vi "MOCOAUTOMATION_1.0.vi"() -> ()   [LabVIEW 2009]
uses:
  autostatus.ctl
  DAQGlobal.vi
  global_m.vi
  1608fsdr/Global 3.vi
  Global 2.vi
panel:
  out "GoTo Wavelength":dbl
  out "Waiting on Move":bool
  out "Exposure Time:":dbl
  out "Number of Steps:":dbl
  out "Step Size:":dbl
  out "Min nm":dbl
  out "Max nm":dbl
  in  "Start up Blinking":bool=TRUE
  in  "Delay Before\nread (ms)":u32=50
  out "delay":u16
  out "back_L":bool
  out "Shutter OFF":bool
  out "Shutter ON":bool
  in  "Tab Control":enum32{"Setup", "Operation"}(tab)
  in  "Automation":bool
  in  "Save settings":bool
  in  "Initialize":bool caption="Push at start up"
  in  "Grating, gr/mm":u16(ring)=2 items=["2400", "1800", "1200", "600", "300", "150"]
  in  "Backlash compensation":dbl=10.0 format="%.2f"
  in  "Backlash":bool
  in  "Calibration, nm":dbl=265.0 format="%2.2f"
  in  "Communication port":refnum<visa-resource-name>="COM1"
  out "Shutter":bool
  in  "Sh_OFF":bool
  in  "Sh_ON":bool
  in  "Speed_set":bool
  in  "Speed":dbl=50.0 format="%.3f"
  in  "stop 2":bool
  in  "fs":bool
  in  "bs":bool
  in  "Wavelength, nm":dbl=10.0 format="%.2f"
  in  "GoTo":bool
  in  "Destination Wavelength":dbl=500.0 format="%.2f"
  out "Present Wavelength":dbl format="%.2f"
  out "move done":bool
  out "string 2":string="\n"
  in  "return":bool
  in  "String To Write 3":string="Y-1?"
  out "Loop":i32
  in  "write":bool
  out "command sent":string="\n"
  out "writing":bool
  in  "stop":bool
  out "read string":string="\n"
  # "Backlash \nCompensation, nm"
  # "nm"
  # "Wavelength"
  # "nm"
  # "Move Wavelength"
  # "nm"
  # "nm/sec"
  # "Shutter"
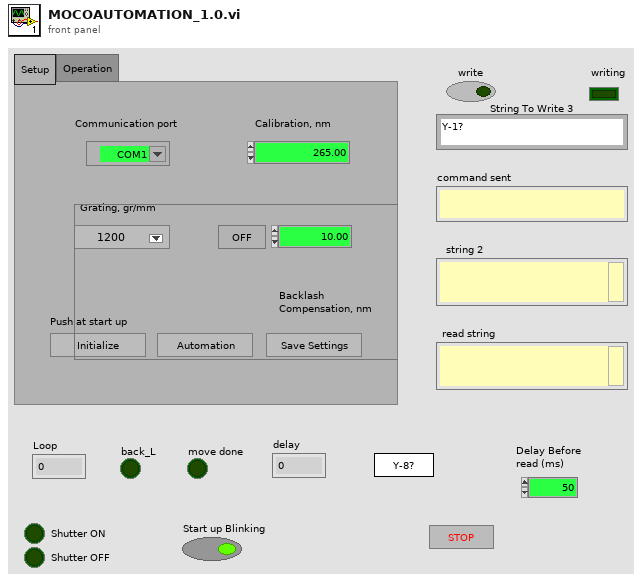
[diagram p1: front panel]
types:
  T1 = enum16{"open", "replace", "create", "open or create", "replace or create", "replace or create with confirmation"}
  T2 = typedef "autostatus.ctl" = enum16{"Default", "Initilize Wavelength", "Shutter Open", "Photodiode Aquire", "Take Img", "Wait Exposure Time", "Photodiode Off", "Shutter Close", "Acquire Dark", "Next Wavelength"}
  T3 = cluster{"Max nm":dbl, "Min nm":dbl, "Step Size:":dbl, "Number of Steps:":dbl, "Exposure Time:":dbl, "Regulation:":bool, "Temperature:":dbl, "Wait_For_Temp:":bool}
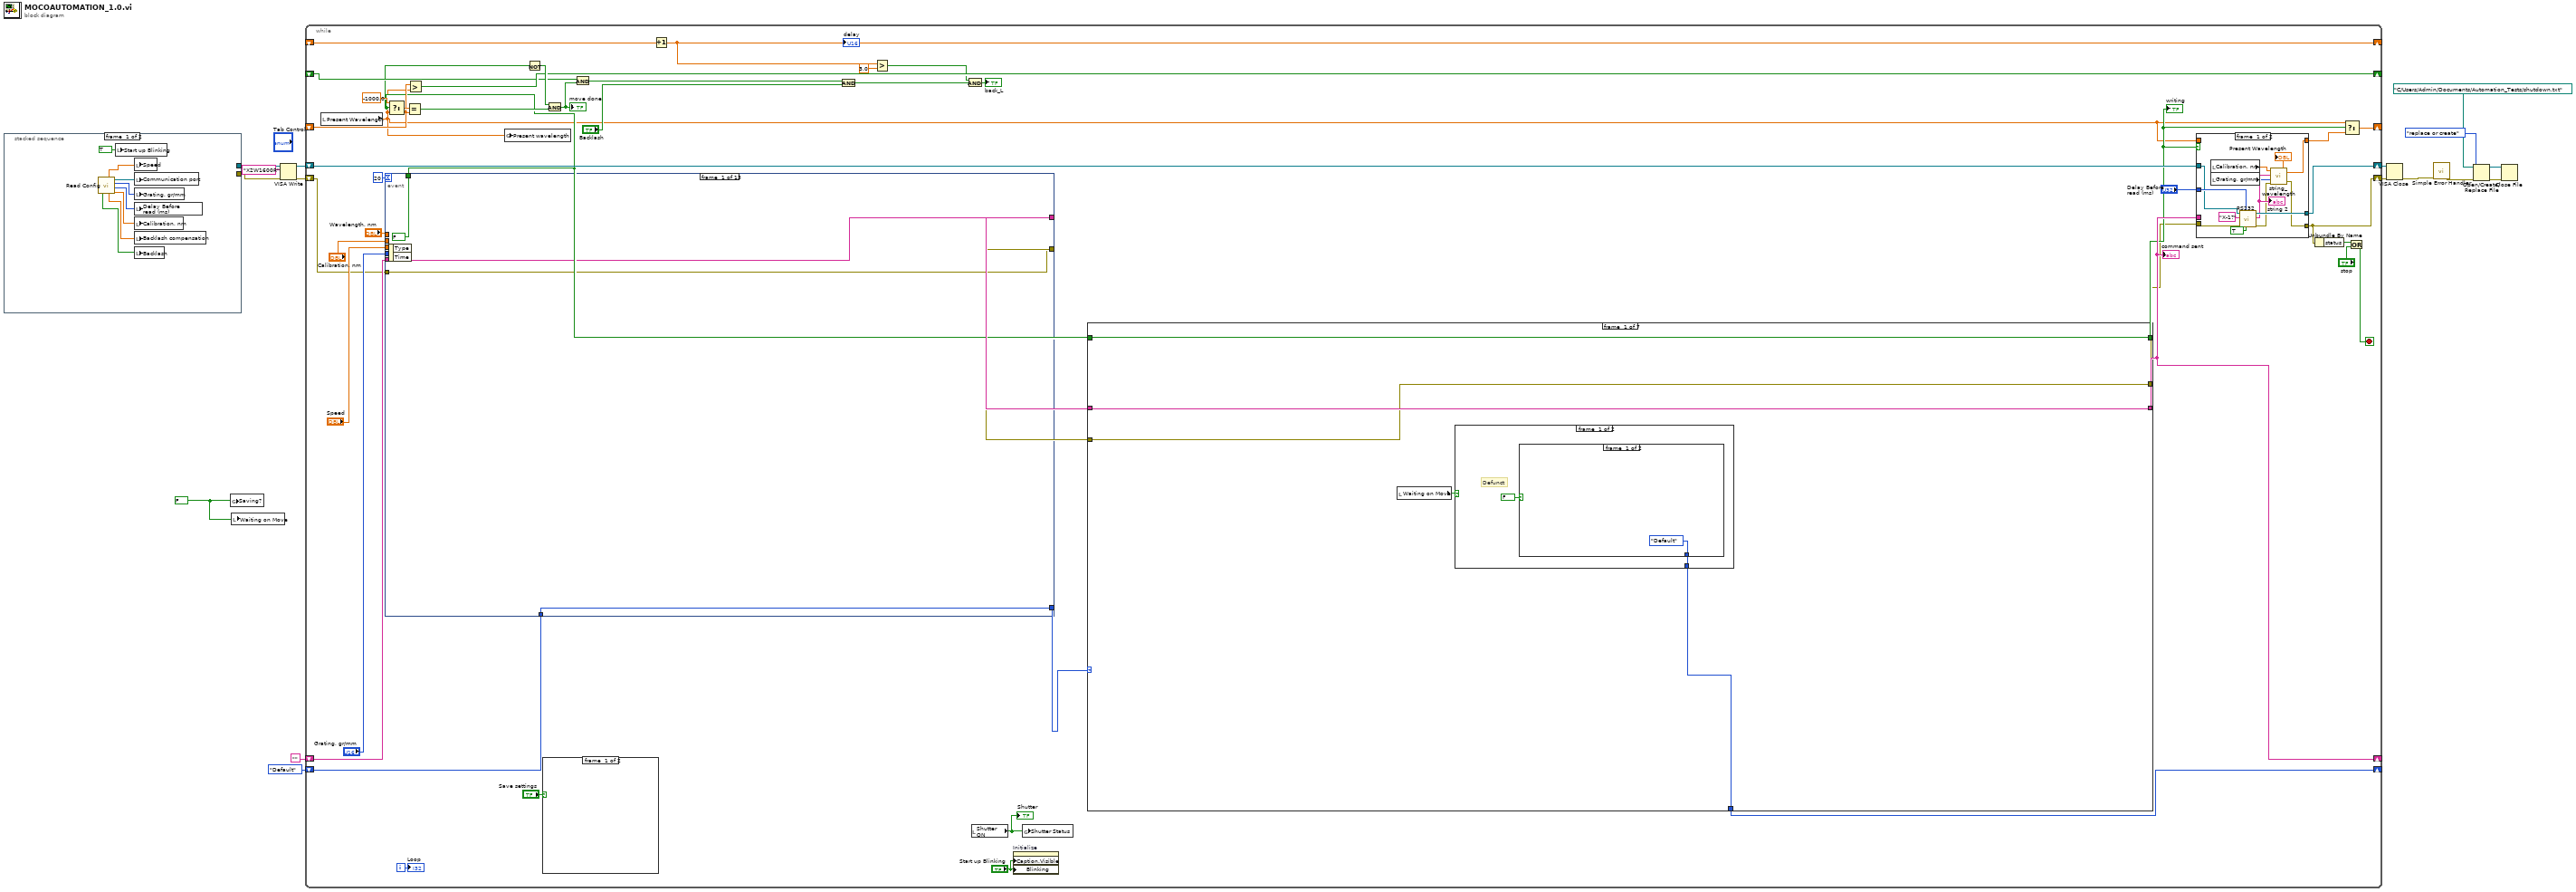
[diagram p0: block diagram]
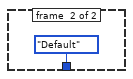
[diagram p2: hidden frame]
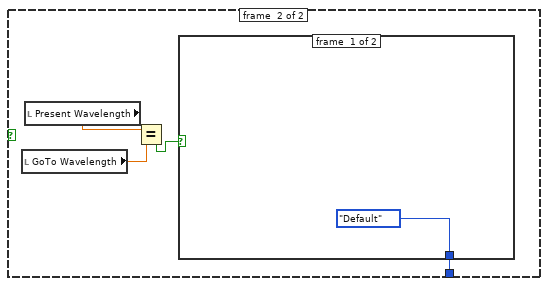
[diagram p3: hidden frame]
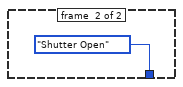
[diagram p4: hidden frame]
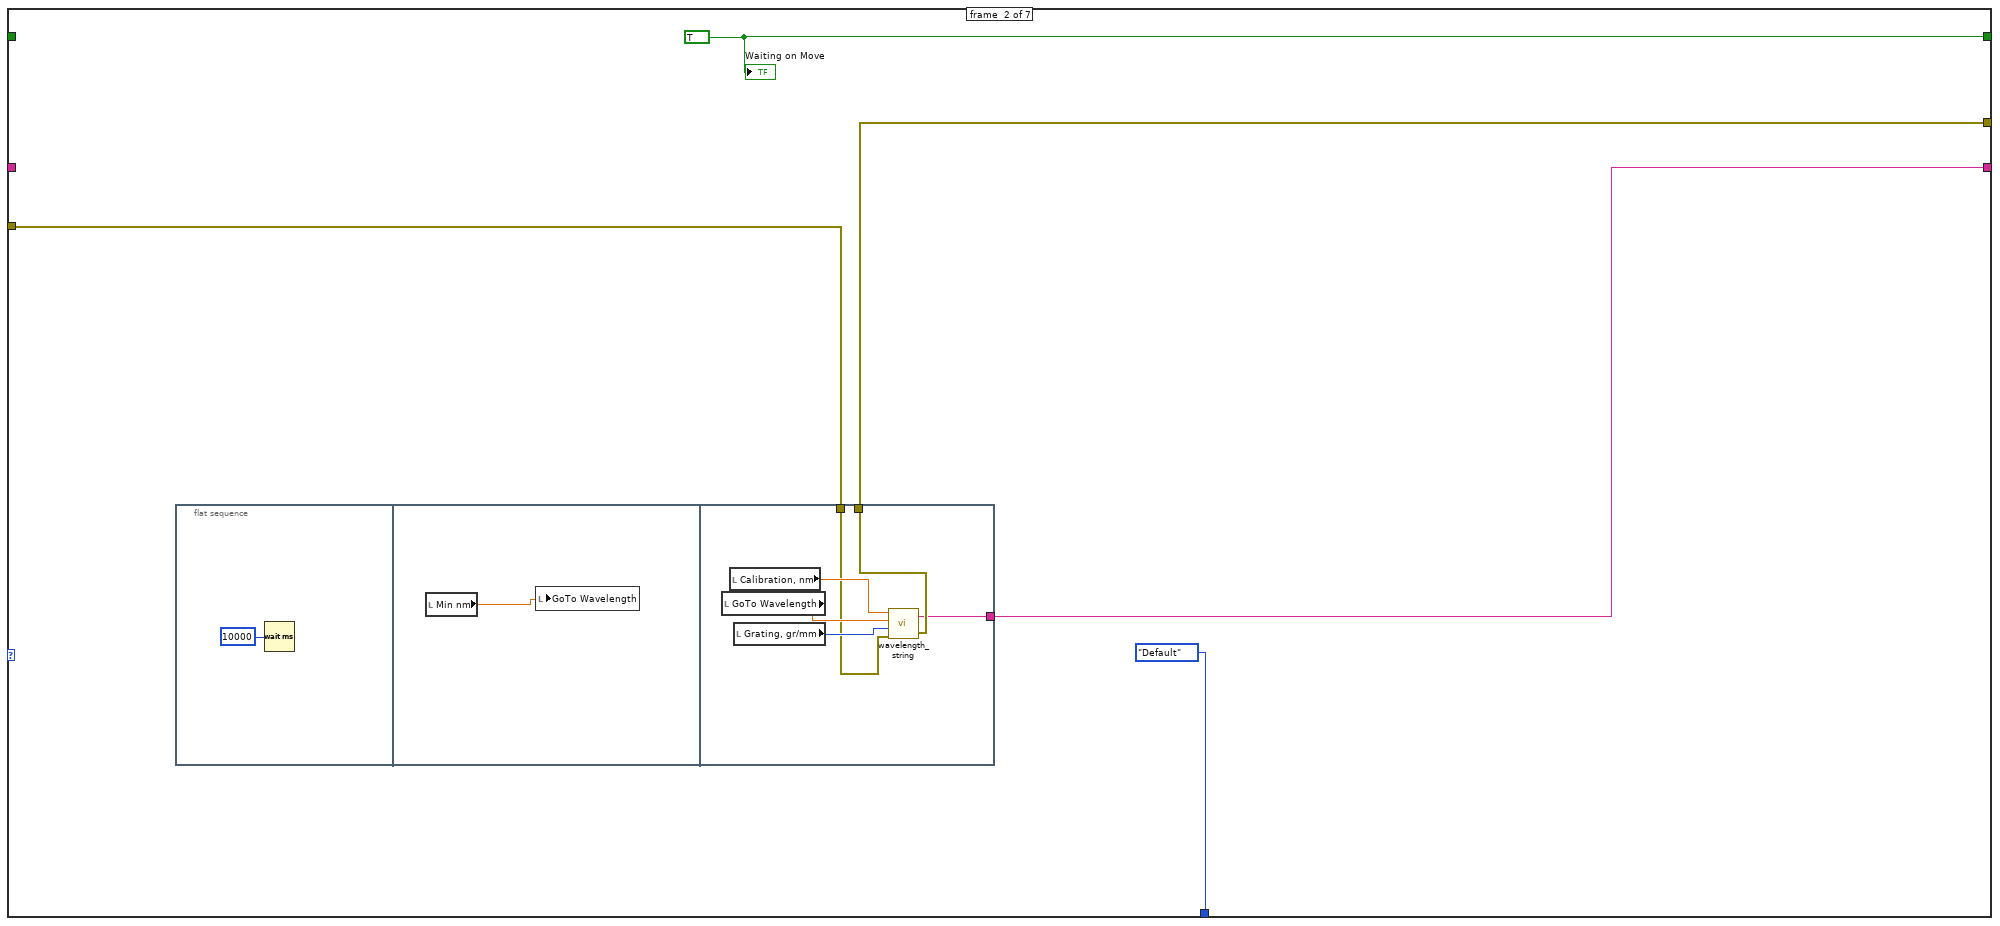
[diagram p5: hidden frame]
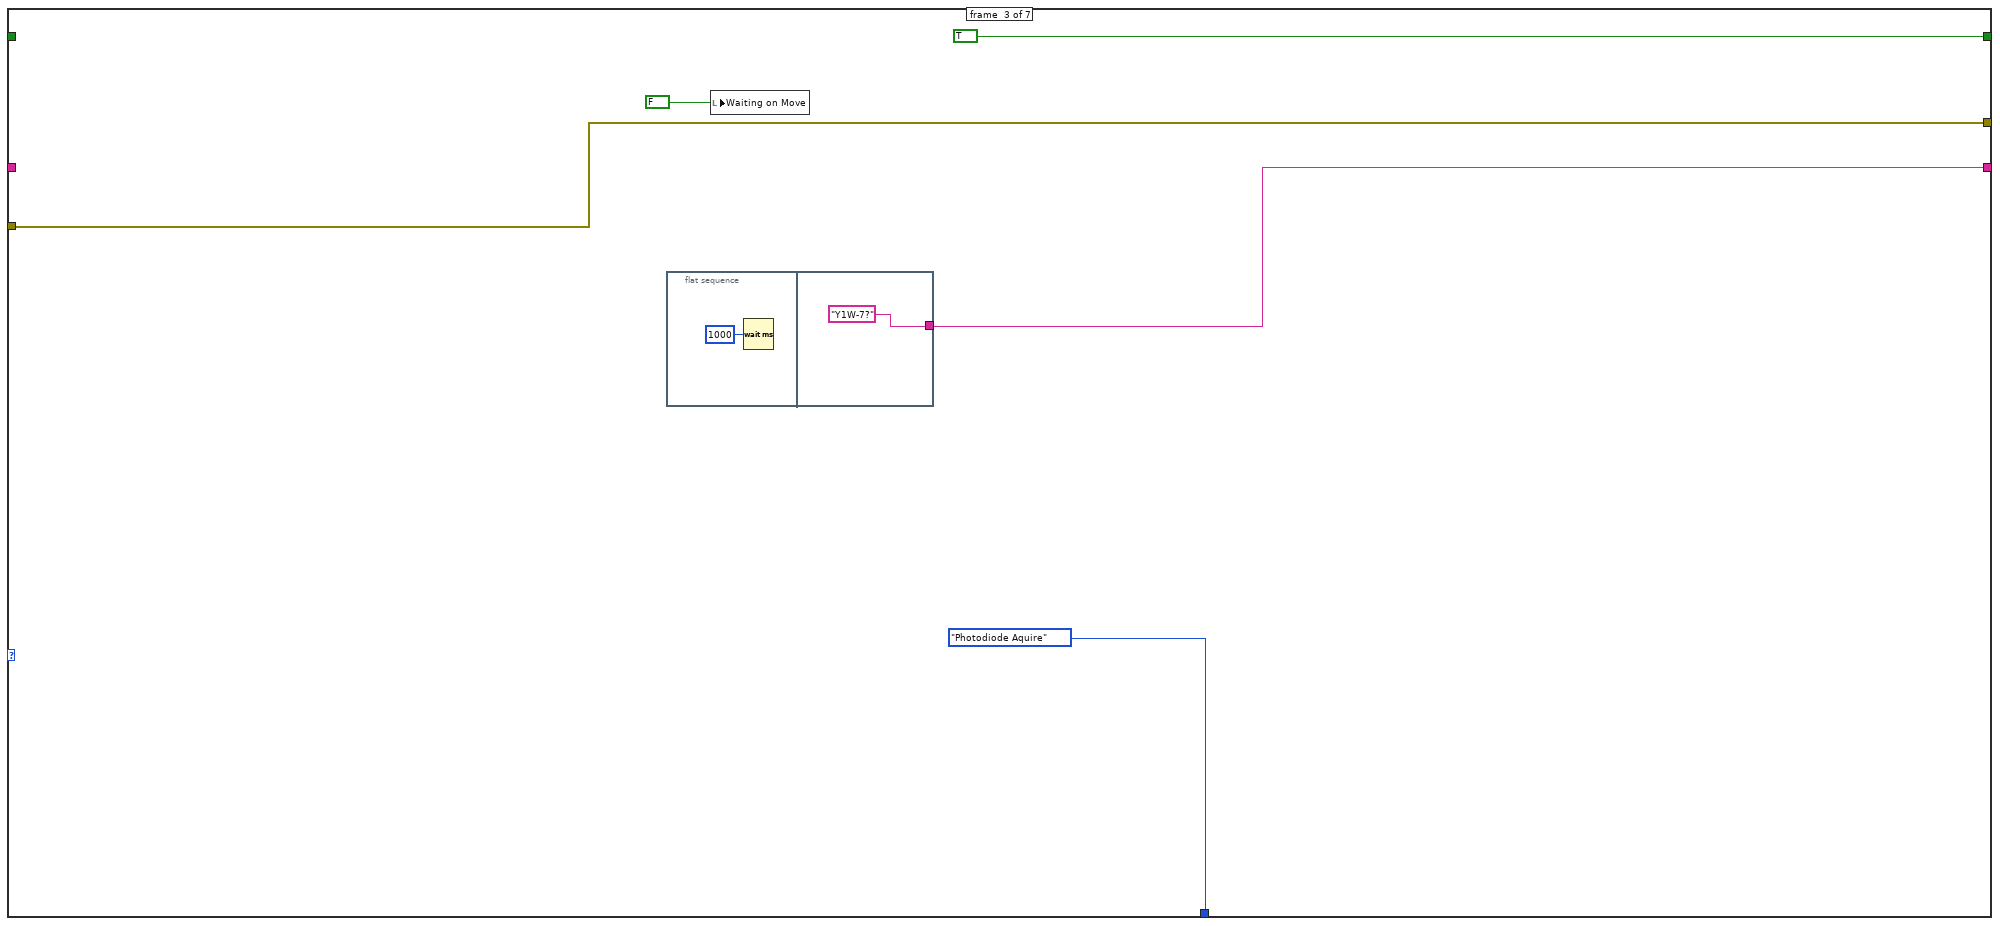
[diagram p6: hidden frame]
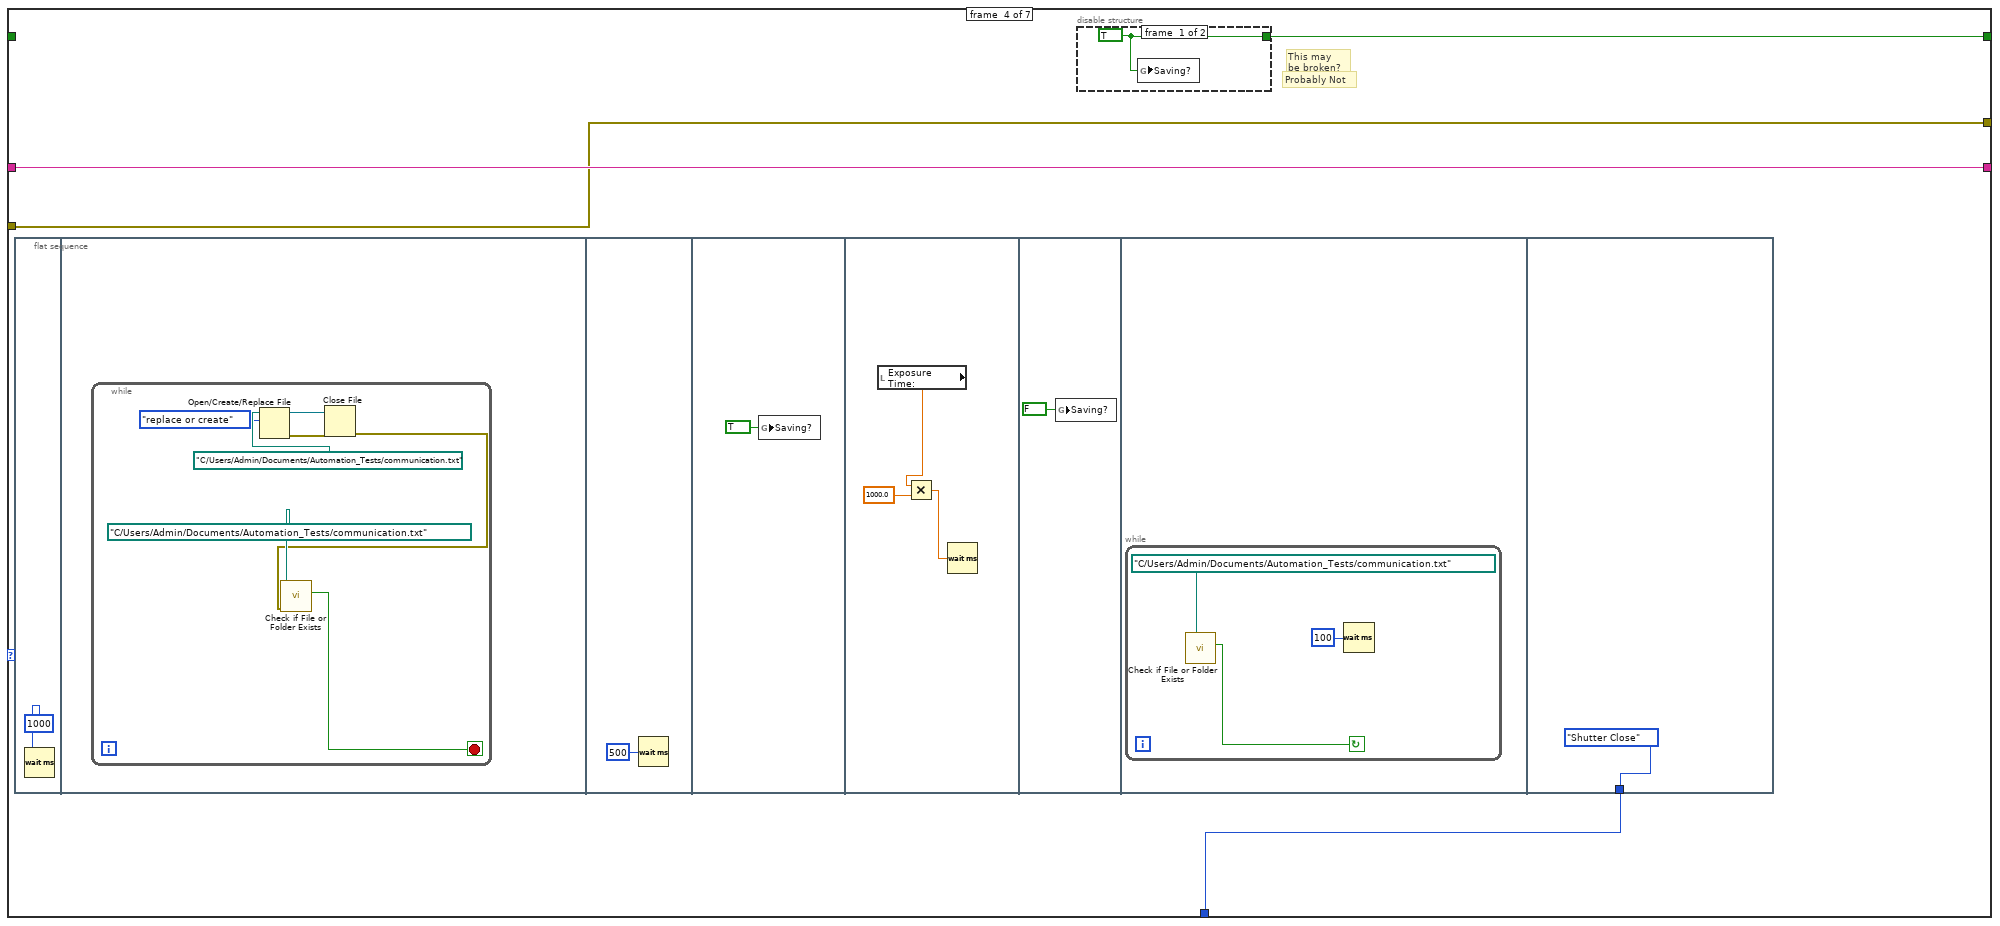
[diagram p7: hidden frame]
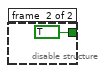
[diagram p8: hidden frame]
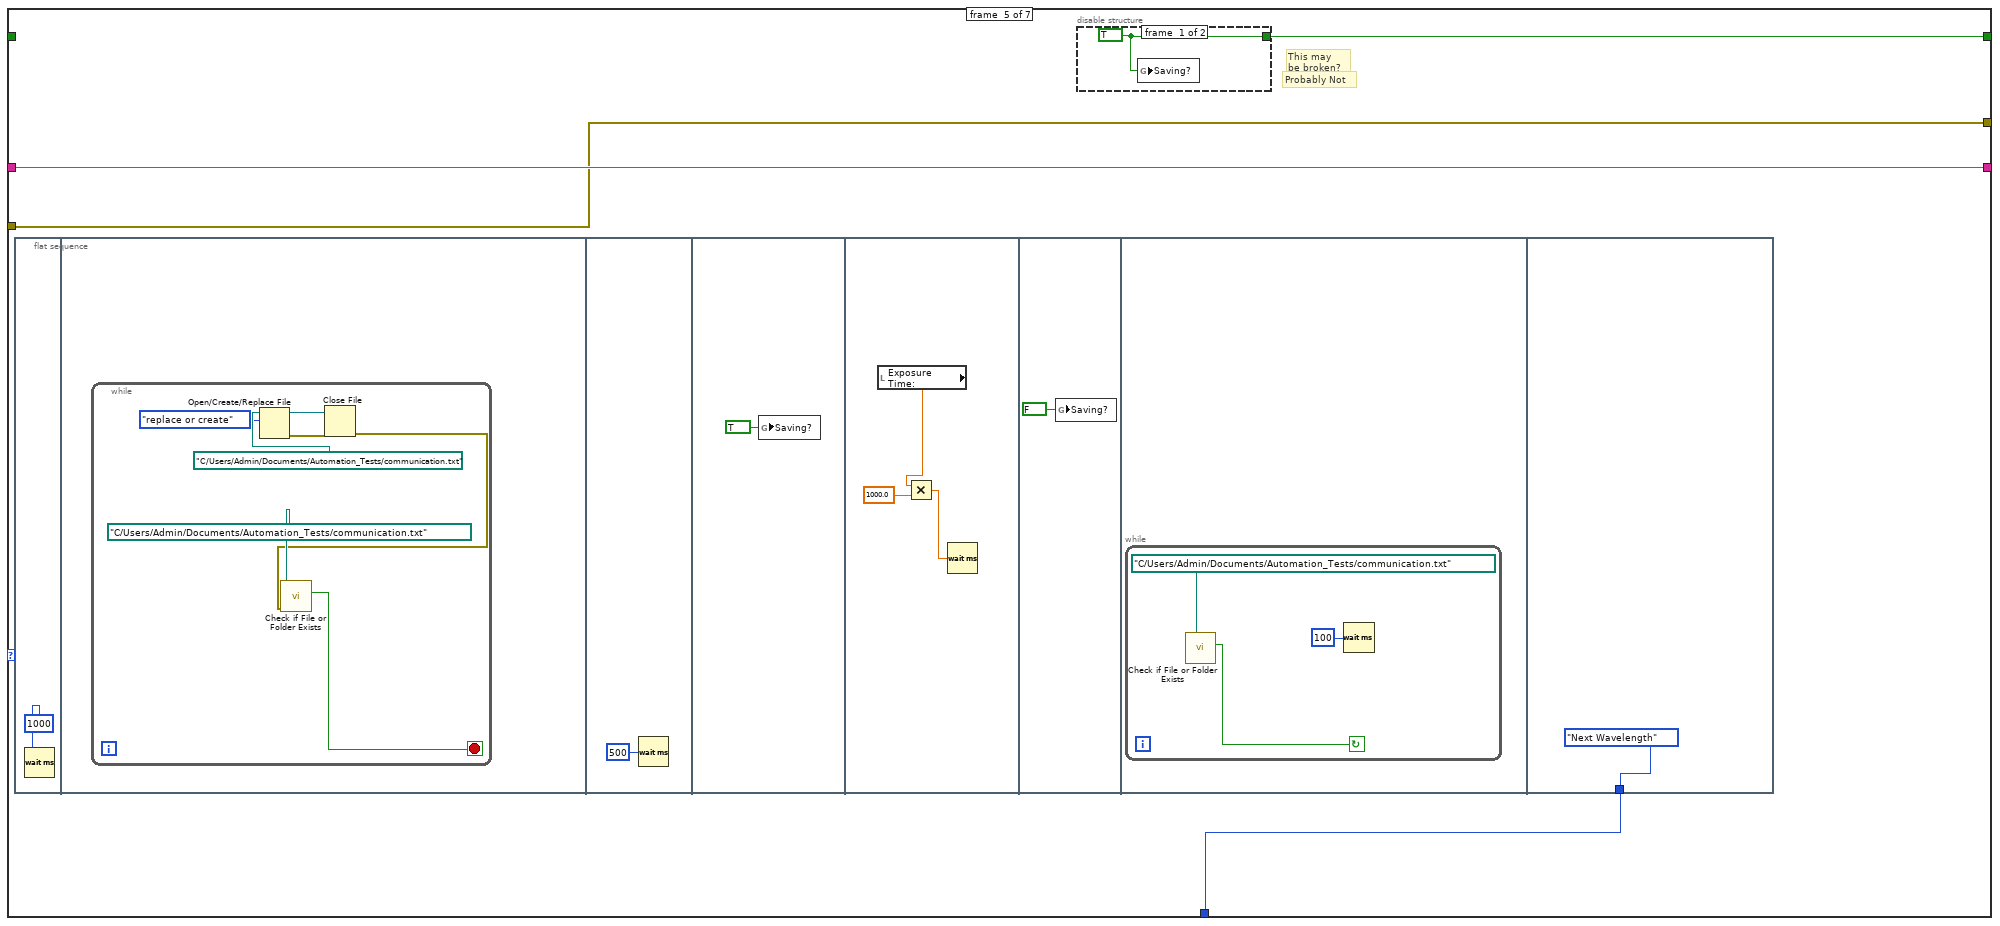
[diagram p9: hidden frame]
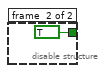
[diagram p10: hidden frame]
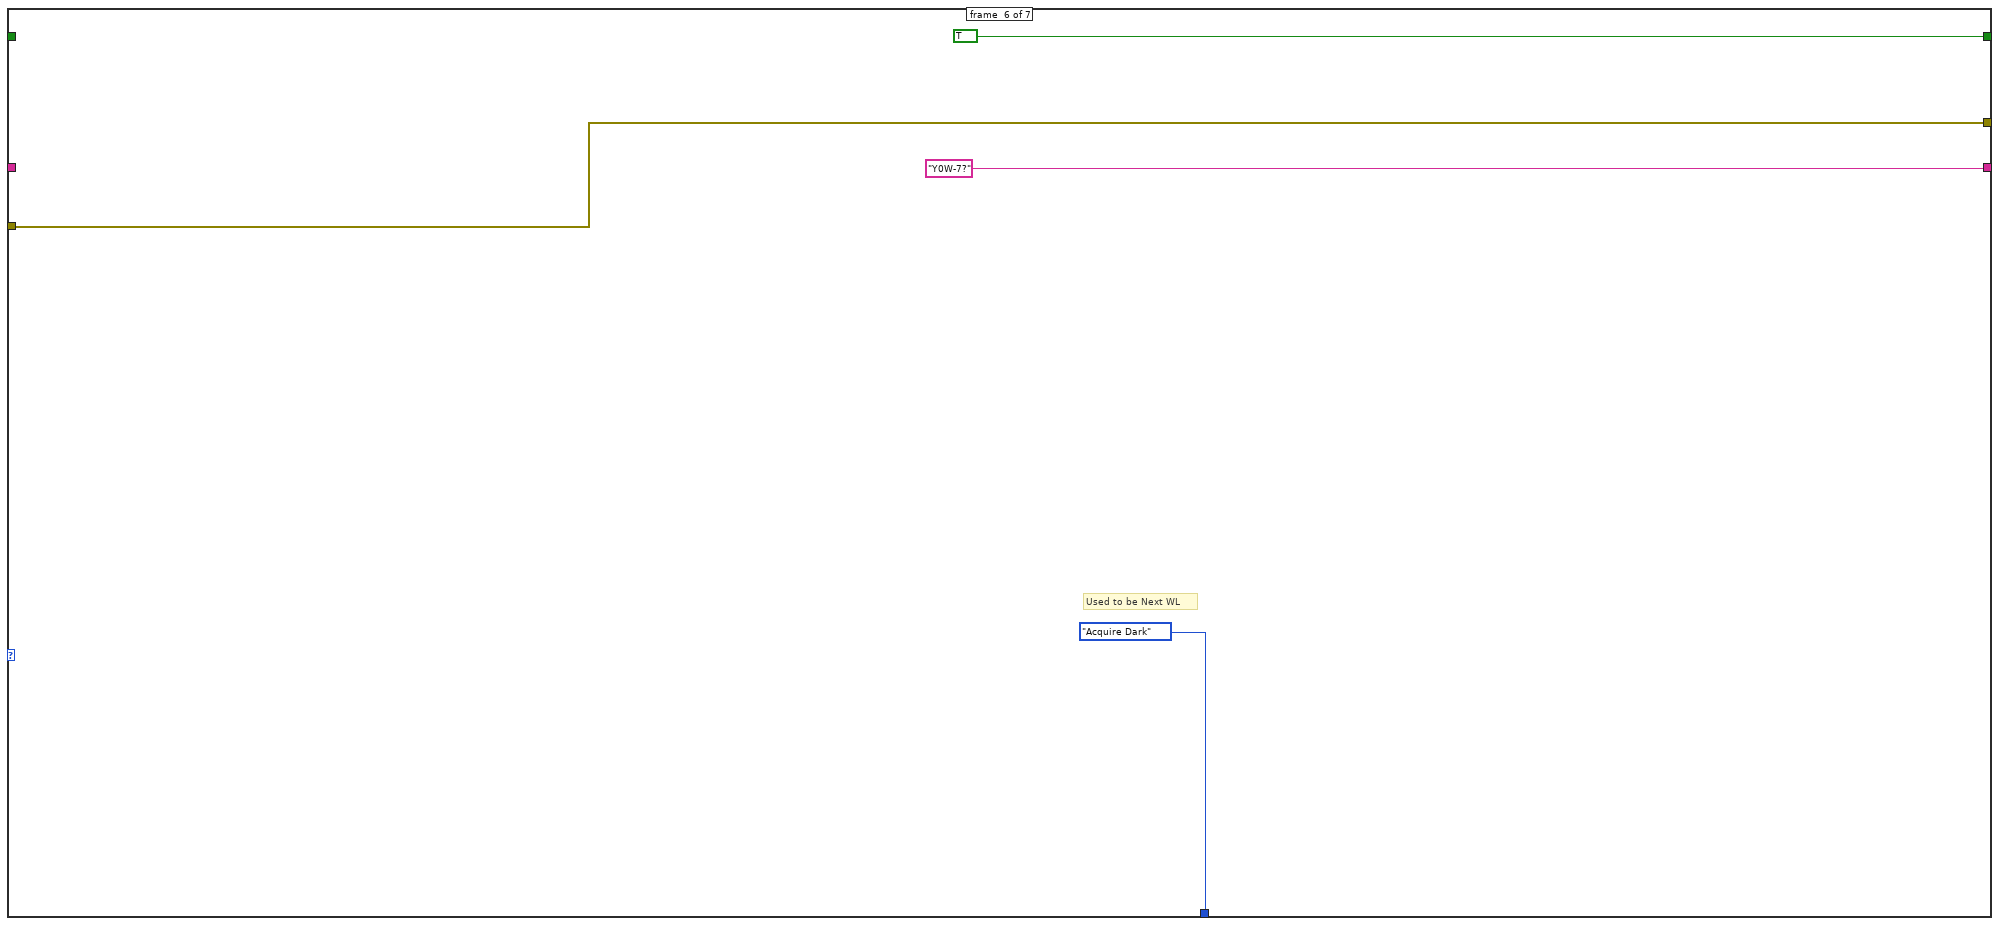
[diagram p11: hidden frame]
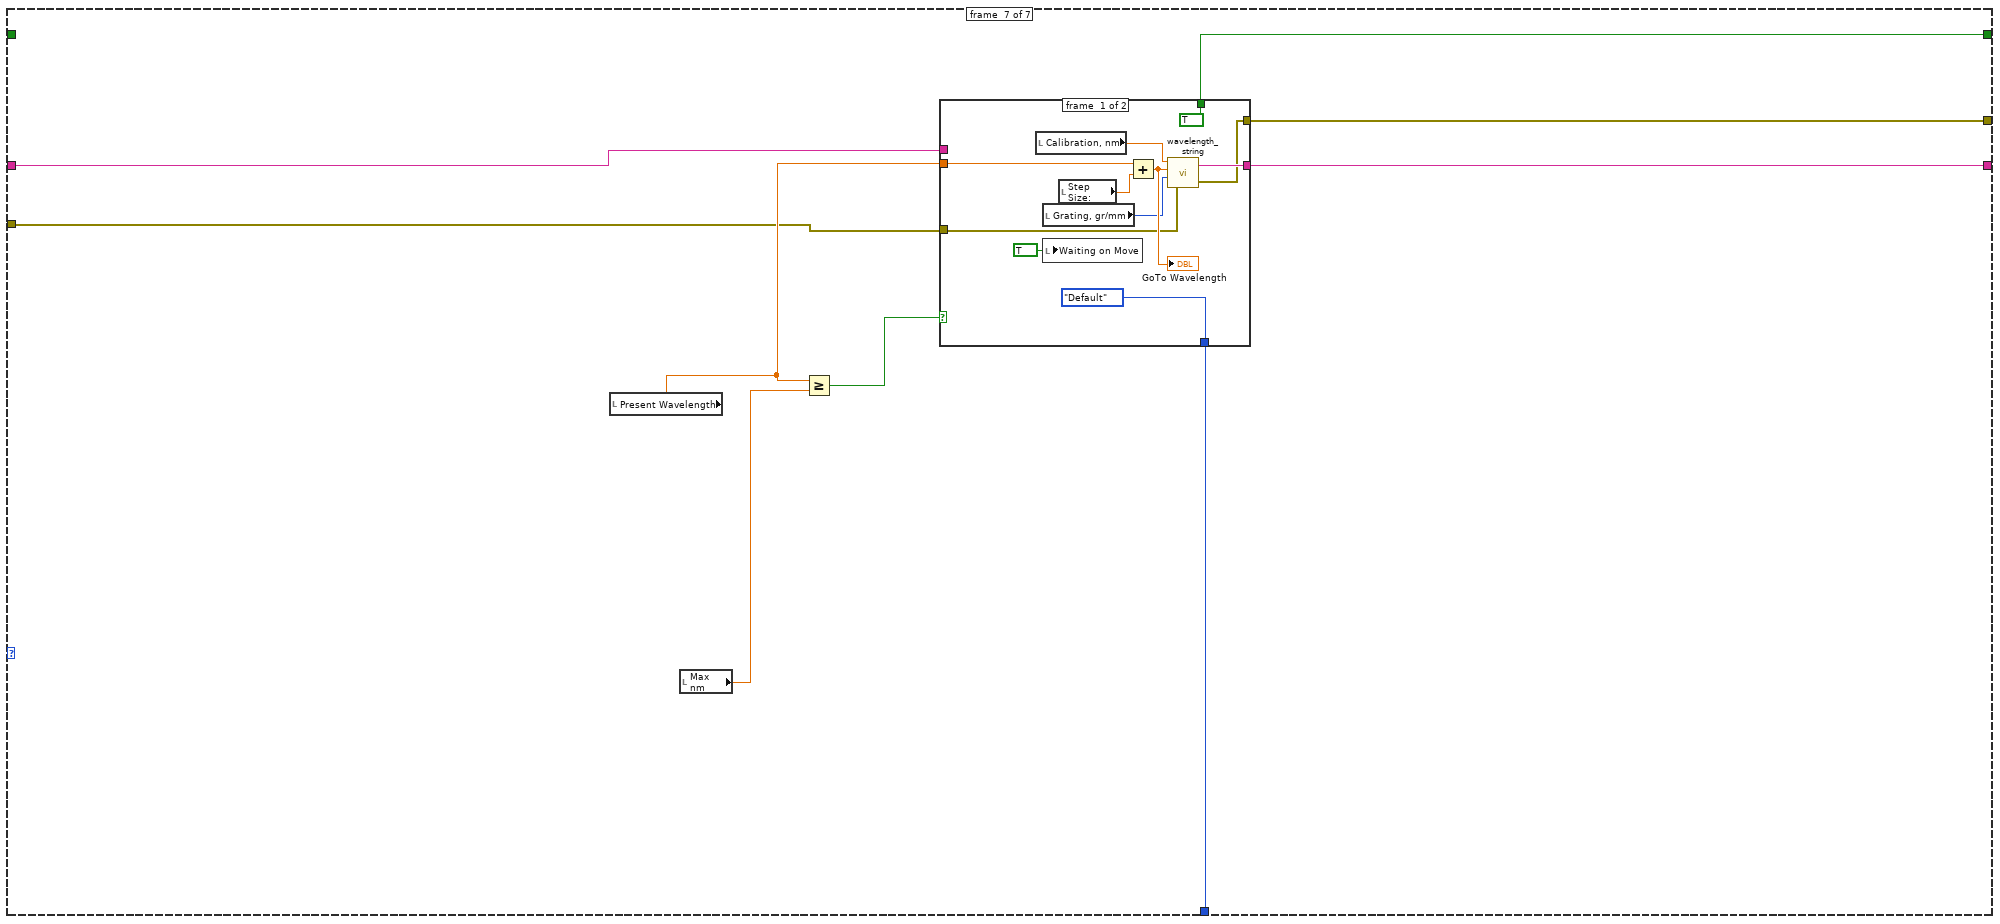
[diagram p12: hidden frame]
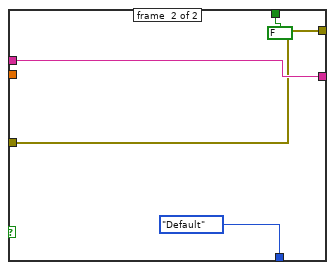
[diagram p13: hidden frame]
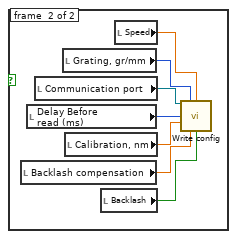
[diagram p14: hidden frame]
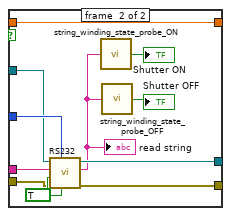
[diagram p15: hidden frame]
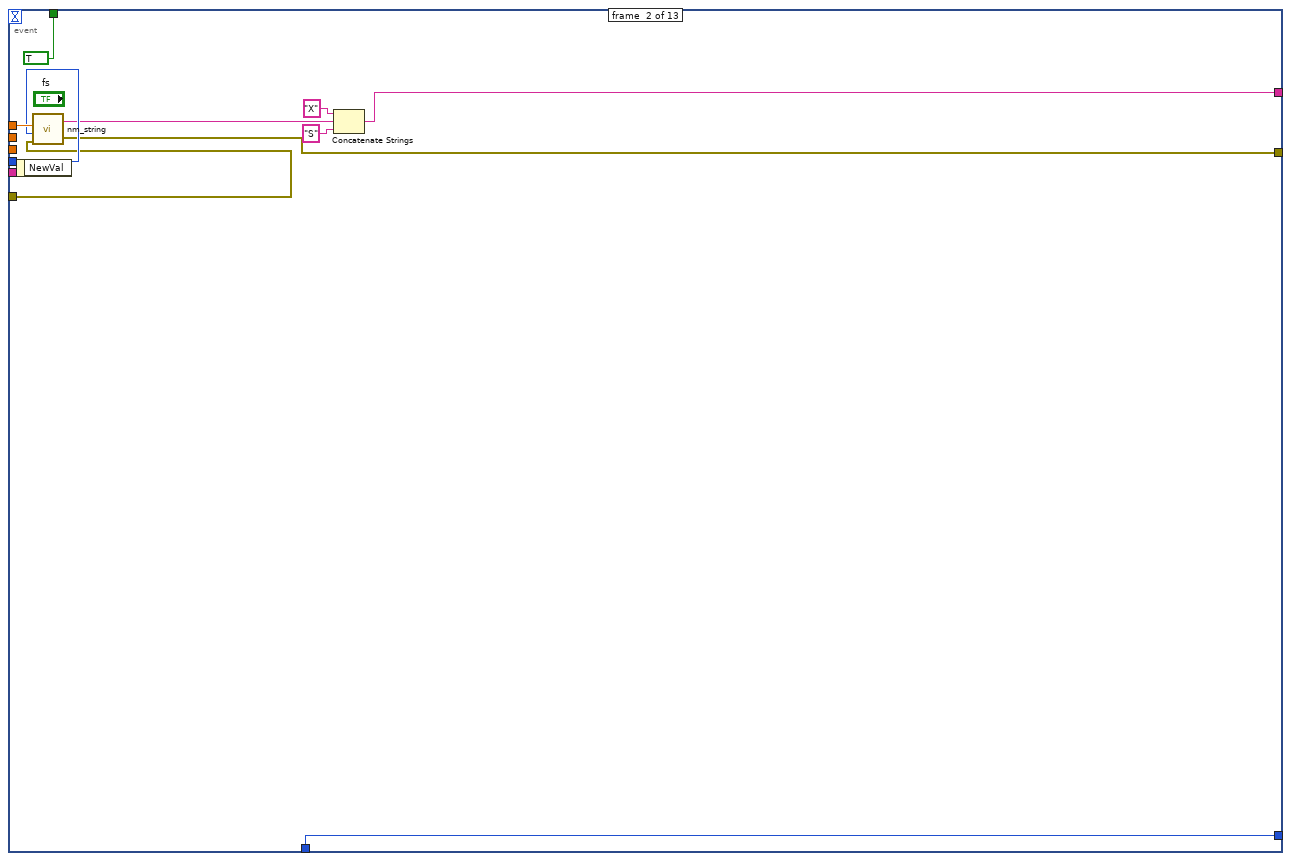
[diagram p16: hidden frame]
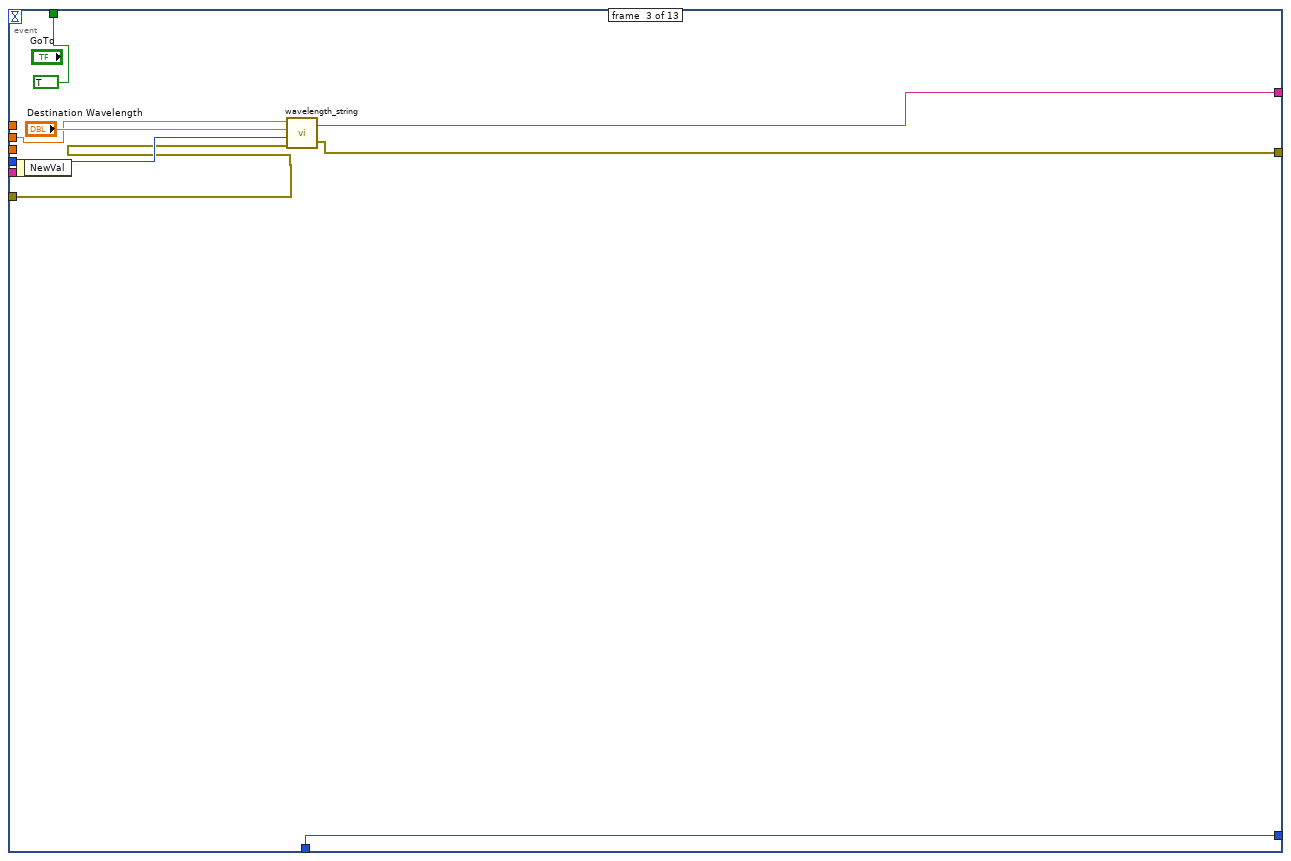
[diagram p17: hidden frame]
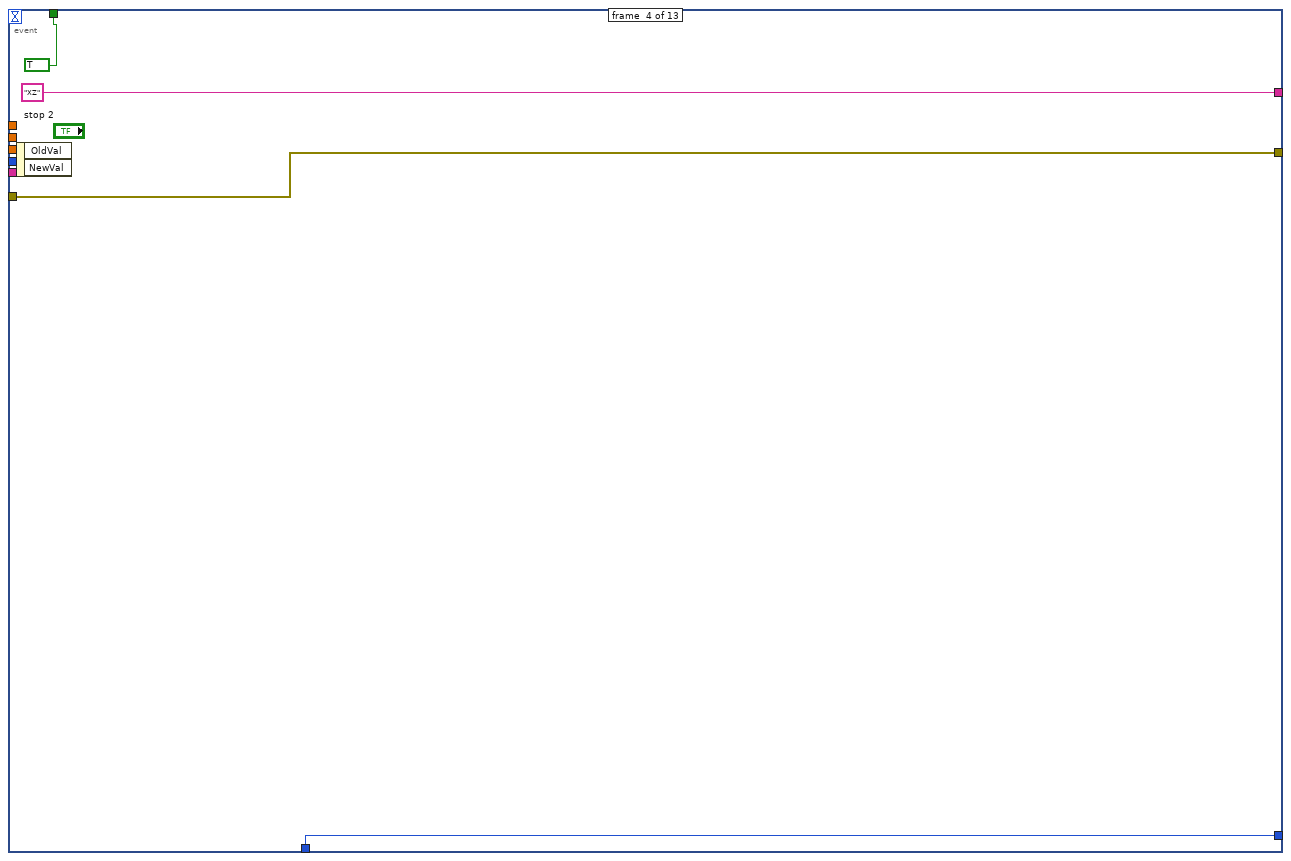
[diagram p18: hidden frame]
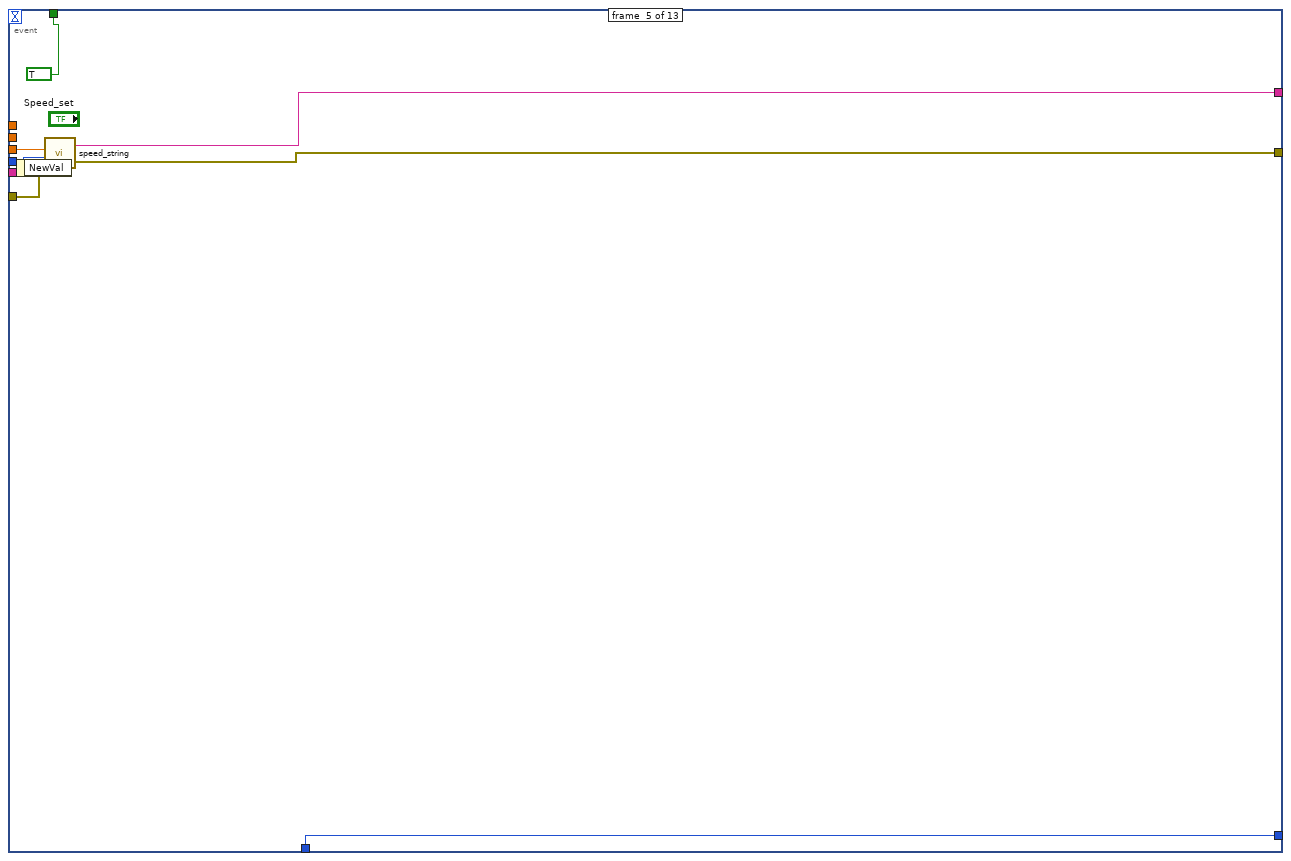
[diagram p19: hidden frame]
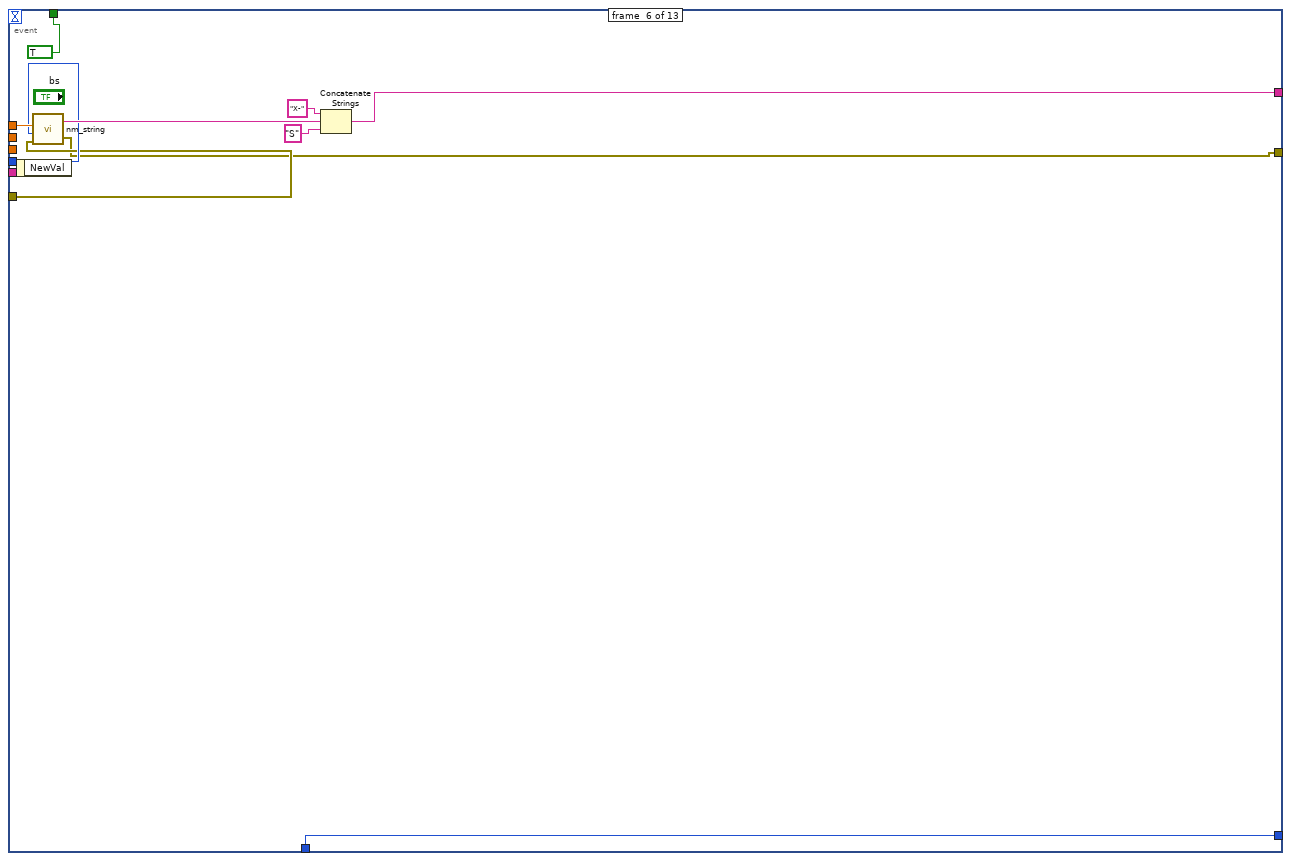
[diagram p20: hidden frame]
diagram:
  w8 = FALSE ("Waiting on Move")
  n1 = stacked-sequence {
    tunnel: [_ w26] -> w13
    tunnel: [_ w25] -> w12
    frame #0 {
      n2 = call "Read Config.vi"() -> ("Backlash"=w17:bool, "Speed"=w20:dbl, "Backlash compensation"=w18:dbl, "VISA resource name"=w21:refnum<visa-resource-name>, "Grating, gr/mm"=w22:u16, "Delay Before read (ms)"=w23:u32, "Calibration, nm"=w19:dbl)  [unwired: 1 in]
      n3 = local write "Start up Blinking"(TRUE ("Start up Blinking")) -> ()
      n4 = local write "Speed"(w20) -> ()
      n5 = local write "Communication port"(w21) -> ()
      n6 = local write "Grating, gr/mm"(w22) -> ()
      n7 = local write "Delay Before\nread (ms)"(w23) -> ()
      n8 = local write "Calibration, nm"(w19) -> ()
      n9 = local write "Backlash compensation"(w18) -> ()
      n10 = local write "Backlash"(w17) -> ()
    }
    frame #1 {
      n11 = global write "global_m.vi" "VISA resource name"("Communication port") -> ()
      n12 = call "RS232_initial.vi"("baud rate"=u32 9600, "VISA resource name"="Communication port") -> ("error out"=w25:errorcluster, "VISA name out"=w26:refnum<visa-resource-name>)  [unwired: 2 in]
    }
  }
  n13 = global write "DAQGlobal.vi" "Saving?"(w8) -> ()
  n14 = local write "Waiting on Move"(w8) -> ()
  n15 = VISA Write(VISA resource name=w13, write buffer="X2W1600R", error in (no error)=w12) -> (VISA resource name out=w15:refnum<visa-resource-name>, error out=w14:errorcluster)  [unwired: 1 out]
  n16 = while {
    shift-right: [w48] -> _
    shift-left: _ -> [w50]
    shift-right: [w35] -> _
    shift-left: _ -> [w58]
    shift-right: [w53] -> _
    shift-left: _ -> [w52]
    shift-right: [w42] -> _
    shift-left: "" -> [w69]
    shift-right: [w40] -> _
    shift-left: autostatus."Default" ("Auto Status") -> [w39]
    shift-right: [w36] -> w7
    shift-left: w14 -> [w30]
    shift-right: [w37] -> w6
    shift-left: w15 -> [w44]
    i -> [w68]
    stop <- w61 stop-if-true
    n17 = local read "Present Wavelength"() -> (w32:dbl)
    n18 = event shown="[10] \"Automation\": Value Change" {
      selector: _ -> [_ _ _ _ _ _ _ _ _ _ _ _ _]
      dyn-events: _ -> [_ _ _ _ _ _ _ _ _ _ _ _ _]
      timeout: 20 -> [_ _ _ _ _ _ _ _ _ _ _ _ _]
      tunnel: "Wavelength, nm" -> [_ w229 _ _ _ w254 _ _ _ _ _ _ _]
      tunnel: "Calibration, nm" -> [_ _ w234 _ _ _ _ _ _ _ _ _ _]
      tunnel: "Speed" -> [_ _ _ _ w248 _ w266 _ _ _ _ _ _]
      tunnel: "Grating, gr/mm" -> [_ w228 w236 _ w247 w253 w265 _ _ w284 _ _ _]
      tunnel: w69 -> [w217 _ _ _ _ _ _ _ _ _ w286 _ _]
      tunnel: [w217 w224 w235 "XZ" ("Wavelength_String") w246 w255 w267 "Y1W-7?" ("nm_String") "Y0W-7?" ("nm_String") "X-1?" ("nm_String") w286 "X-8?" ("nm_String") "String To Write 3"] -> w43
      tunnel: [FALSE ("writing") TRUE ("writing") TRUE ("writing") TRUE ("writing") TRUE ("writing") TRUE ("writing") TRUE ("writing") TRUE ("writing") TRUE ("writing") TRUE ("writing") FALSE ("writing") TRUE ("writing") TRUE ("writing")] -> w41
      tunnel: w39 -> [w218 w222 w232 w239 w244 w251 w261 w271 w275 w279 w288 w334 w338]
      tunnel: [w218 w222 w232 w239 w244 w251 w261 w271 w275 w279 w287 w334 w338] -> w38
      tunnel: w30 -> [w216 w221 w231 w238 w243 w250 w260 w270 w274 w278 w285 w333 w337]
      tunnel: [w216 w220 w230 w238 w242 w249 w259 w270 w274 w278 w285 w333 w337] -> w31
      event #0 {
        n19 = event-data() -> ()  [unwired: 1 in, 2 out]
      }
      event #1 {
        n20 = event-data() -> ()  [unwired: 1 in, 1 out]
        n21 = call "nm_string.vi"("error in (no error)"=w221, "Grating, gr/mm"=w228, "Wavelength, nm"=w229) -> ("error out"=w220:errorcluster, "nm_String"=w227:string)  [unwired: 1 in]
        n22 = Concatenate Strings("X" ("string"), w227, "S" ("string")) -> (w224:string)
      }
      event #2 {
        n23 = event-data() -> ()  [unwired: 1 in, 1 out]
        n24 = call "wavelength_string.vi"("error in (no error)"=w231, "Grating, gr/mm"=w236, "Destination Wavelength"="Destination Wavelength", "Calibration, nm"=w234) -> ("error out"=w230:errorcluster, "Wavelength_String"=w235:string)
      }
      event #3 {
        n25 = event-data() -> ()  [unwired: 1 in, 2 out]
      }
      event #4 {
        n26 = event-data() -> ()  [unwired: 1 in, 1 out]
        n27 = call "speed_string.vi"("error in (no error)"=w243, "Grating, gr/mm"=w247, "Speed"=w248) -> ("error out"=w242:errorcluster, "nm_String"=w246:string)  [unwired: 1 in]
      }
      event #5 {
        n28 = event-data() -> ()  [unwired: 1 in, 1 out]
        n29 = call "nm_string.vi"("error in (no error)"=w250, "Grating, gr/mm"=w253, "Wavelength, nm"=w254) -> ("error out"=w249:errorcluster, "nm_String"=w258:string)  [unwired: 1 in]
        n30 = Concatenate Strings("X-" ("string"), w258, "S" ("string")) -> (w255:string)
      }
      event #6 {
        n31 = event-data() -> ("NewVal"=w264:bool)  [unwired: 1 in]
        n32 = call "speed_string.vi"("error in (no error)"=w260, "Grating, gr/mm"=w265, "Speed"=w266) -> ("error out"=w259:errorcluster, "nm_String"=w267:string)  [unwired: 1 in]
        n33 = call "initialize.vi"() -> ()  [unwired: 3 in]
        n34 = case shown="True" w264 {
          selector: w264 -> [_ w269]
          frame #0 {
          }
          frame #1 {
            n35 = Not(x=w269) -> (.not. x?=w268:bool)
            n36 = local write "Start up Blinking"(w268) -> ()
          }
        }
        n37 = local write "delay"(u16 1 ("delay")) -> ()
      }
      event #7 {
        n38 = event-data() -> ()  [unwired: 1 in, 1 out]
      }
      event #8 {
        n39 = event-data() -> ()  [unwired: 1 in, 1 out]
      }
      event #9 {
        n40 = event-data() -> ()  [unwired: 1 in, 2 out]
        n41 = local write "delay"(u16 1 ("delay")) -> ()
        n42 = call "backlash_move.vi"("Grating, gr/mm"=w284, "Wavelength, nm"="Backlash compensation") -> ()  [unwired: 3 in]
      }
      event #10 {
        n43 = event-data() -> ()  [unwired: 1 in, 1 out]
        n44 = call "mocoautomation.vi"() -> ("Automation Settings"=w290:T3, "Canceled?"=w291:bool)  [unwired: 1 in]
        n45 = case shown="False" w291 {
          tunnel: w290 -> [w310 _]
          tunnel: w288 -> [_ _]
          tunnel: [autostatus."Initilize Wavelength" ("Auto Status") autostatus."Default" ("Auto Status")] -> w287
          frame #0 {
            w325 = "\r\n"
            n46 = local read "Min nm"() -> (w320:dbl)
            n47 = local read "Max nm"() -> (w319:dbl)
            n48 = local read "Exposure Time:"() -> (w321:dbl)
            n49 = local read "Step Size:"() -> (w318:dbl)
            n50 = Unbundle(w310) -> ("Max nm"=→"Max nm":dbl, "Min nm"=→"Min nm":dbl, "Step Size:"=→"Step Size:":dbl, "Number of Steps:"=→"Number of Steps:":dbl, "Exposure Time:"=→"Exposure Time:":dbl, "Regulation:"=w302:bool, "Temperature:"=w299:dbl, "Wait_For_Temp:"=w292:bool)
            n51 = Boolean To (0,1)(Boolean=w302) -> (0, 1=w301:i16)
            n52 = Open/Create/Replace File(file path (use dialog)=path "C:/Users/Admin/Documents/MocoAutomation/CCDrunfile.bat", operation (0:open)=T1."replace or create") -> (refnum out=w326:refnum<file>, error out=w327:errorcluster)  [unwired: 4 in, 1 out]
            n53 = Number To Decimal String(number=w320) -> (decimal integer string=w297:string)  [unwired: 1 in]
            n54 = Number To Decimal String(number=w319) -> (decimal integer string=w296:string)  [unwired: 1 in]
            n55 = Number To Decimal String(number=w321) -> (decimal integer string=w303:string)  [unwired: 1 in]
            n56 = Number To Decimal String(number=w318) -> (decimal integer string=w294:string)  [unwired: 1 in]
            n57 = Number To Decimal String(number=w301) -> (decimal integer string=w300:string)  [unwired: 1 in]
            n58 = Number To Decimal String(number=w299) -> (decimal integer string=w298:string)  [unwired: 1 in]
            n59 = call <vilib>:"Space Constant.vi"() -> ("String"=w295:string)
            n60 = Concatenate Strings("CCDautomation.exe" ("string"), w295, w303, w295, w300, w295, w298, w295, w297, w295, w296, w295, w294) -> (w311:string)
            n61 = Concatenate Strings("@ECHO OFF" ("string"), w325, "cd C:\\Users\\Admin\\Documents\\MoCoAutomation" ("string"), w325, w311, w325, "exit" ("string")) -> (w317:string)
            n62 = Write to Text File(file (use dialog)=w326, text=w317, error in=w327) -> (refnum out=w313:refnum<file>, error out=w314:errorcluster)  [unwired: 1 in, 1 out]
            n63 = Close File(refnum=w313, error in=w314) -> (error out=w312:errorcluster)  [unwired: 1 out]
            n64 = call <vilib>:"System Exec.vi"("wait until completion? (T)"=FALSE, "error in (no error)"=w312, "working directory"=path "C:/Users/Admin/Documents/MoCoAutomation", "command line"="CCDrunfile.bat") -> ()  [unwired: 4 in, 4 out]
            n65 = case shown="True" w292 {
              frame #0 {
              }
              frame #1 {
                n66 = Wait (ms)(milliseconds to wait=u32 300000) -> ()  [unwired: 1 out]
              }
            }
          }
          frame #1 {
          }
        }
      }
      event #11 {
        n67 = event-data() -> ()  [unwired: 1 in, 1 out]
      }
      event #12 {
        n68 = event-data() -> ()  [unwired: 1 in, 2 out]
      }
    }
    n69 = Select(t=-1000.0, s=w41, f=w32) -> (s? t:f=w59:dbl)
    n70 = Equal?(x=w59, y=w58) -> (x = y?=w56:bool)
    n71 = Greater?(x=w58, y=w32) -> (0:w53:bool)
    n72 = global write "Global 2.vi" "Present wavelength"(w32) -> ()
    n73 = Not(x=w41) -> (.not. x?=w57:bool)
    n74 = case shown="True" "Save settings" {
      frame #0 {
      }
      frame #1 {
        n75 = local read "Backlash compensation"() -> (w187:dbl)
        n76 = local read "Delay Before\nread (ms)"() -> (w189:u32)
        n77 = local read "Communication port"() -> (w190:refnum<visa-resource-name>)
        n78 = local read "Grating, gr/mm"() -> (w191:u16)
        n79 = local read "Calibration, nm"() -> (w188:dbl)
        n80 = local read "Backlash"() -> (w186:bool)
        n81 = local read "Speed"() -> (w192:dbl)
        n82 = call "Write config.vi"("VISA resource name"=w190, "Grating, gr/mm"=w191, "Speed"=w192, "Delay Before read (ms)"=w189, "Calibration, nm"=w188, "Backlash compensation"=w187, "Backlash"=w186) -> ()  [unwired: 9 in]
      }
    }
    n83 = And(x=w57, y=w56) -> (x .and. y?=w51:bool)
    "move done" <- w51
    n84 = And(x=w52, y=w51) -> (x .and. y?=w55:bool)
    n85 = Increment(x=w50) -> (x+1=w48:dbl)
    "delay" <- w48
    n86 = And(x=w55, y="Backlash") -> (x .and. y?=w46:bool)
    n87 = Greater?(x=w48, y=3.0) -> (0:w49:bool)
    n88 = And(x=w49, y=w46) -> (x .and. y?=→"back_L":bool)
    n89 = local read "Shutter ON"() -> (w67:bool)
    "Shutter" <- w67
    n90 = property on="Initialize" class="Bool"("Caption.Visible"="Start up Blinking", "Blinking"="Start up Blinking") -> ()  [unwired: 2 in, 2 out]
    n91 = global write "Global 3.vi" "Shutter Status"(w67) -> ()
    n92 = case shown="\"Photodiode Aquire\"" w38 {
      tunnel: [w79 w90 w103 w113 w137 "Y0W-7?" ("nm_String") w168] -> w42
      tunnel: w43 -> [w79 _ _ w113 w137 _ w165]
      tunnel: w41 -> [w78 _ _ _ _ _ _]
      tunnel: [w78 w94 TRUE ("Waiting on Move") w111 w135 TRUE ("Waiting on Move") w166] -> w33
      tunnel: [w76 autostatus."Default" ("Auto Status") autostatus."Photodiode Aquire" ("Auto Status") w110 w134 autostatus."Acquire Dark" ("Auto Status") w164] -> w40
      tunnel: w31 -> [w75 w92 w104 w112 w136 w158 w163]
      tunnel: [w75 w91 w104 w112 w136 w158 w162] -> w29
      frame #0 {
        n93 = local read "Waiting on Move"() -> (w77:bool)
        n94 = case shown="True" w77 {
          tunnel: [w81 w87] -> w76
          frame #0 {
            # "Defunct"
            n95 = case shown="True" FALSE {
              tunnel: [autostatus."Default" ("Auto Status") autostatus."Default" ("Auto Status")] -> w81
              frame #0 {
              }
              frame #1 {
              }
            }
          }
          frame #1 {
            n96 = local read "GoTo Wavelength"() -> (w85:dbl)
            n97 = local read "Present Wavelength"() -> (w86:dbl)
            n98 = Equal?(x=w86, y=w85) -> (x = y?=w84:bool)
            n99 = case shown="True" w84 {
              tunnel: [autostatus."Default" ("Auto Status") autostatus."Shutter Open" ("Auto Status")] -> w87
              frame #0 {
              }
              frame #1 {
              }
            }
          }
        }
      }
      frame #1 {
        w94 = TRUE ("Waiting on Move")
        n100 = flat-sequence {
          tunnel: w92 -> [w99]
          tunnel: [w98] -> w91
          tunnel: [w97] -> w90
          frame #0 {
            n101 = Wait (ms)(milliseconds to wait=u32 10000) -> ()  [unwired: 1 out]
          }
          frame #1 {
            n102 = local read "Min nm"() -> (w96:dbl)
            n103 = local write "GoTo Wavelength"(w96) -> ()
          }
          frame #2 {
            n104 = local read "GoTo Wavelength"() -> (w100:dbl)
            n105 = local read "Calibration, nm"() -> (w102:dbl)
            n106 = local read "Grating, gr/mm"() -> (w101:u16)
            n107 = call "wavelength_string.vi"("error in (no error)"=w99, "Grating, gr/mm"=w101, "Destination Wavelength"=w100, "Calibration, nm"=w102) -> ("error out"=w98:errorcluster, "Wavelength_String"=w97:string)
          }
        }
        "Waiting on Move" <- w94
      }
      frame #2 {
        n108 = flat-sequence {
          tunnel: ["Y1W-7?" ("nm_String")] -> w103
          frame #0 {
            n109 = Wait (ms)(milliseconds to wait=u32 1000) -> ()  [unwired: 1 out]
          }
          frame #1 {
          }
        }
        n110 = local write "Waiting on Move"(FALSE ("Waiting on Move")) -> ()
      }
      frame #3 {
        # "Probably Not"
        # "This may \nbe broken?"
        n111 = flat-sequence {
          tunnel: [autostatus."Shutter Close" ("Auto Status")] -> w110
          frame #0 {
            n112 = Wait (ms)(milliseconds to wait=u32 1000) -> ()  [unwired: 1 out]
          }
          frame #1 {
            n113 = while {
              stop <- w118 stop-if-true
              n114 = Open/Create/Replace File(file path (use dialog)=path "C:/Users/Admin/Documents/Automation_Tests/communication.txt" ("file (use dialog)"), operation (0:open)=T1."replace or create") -> (refnum out=w122:refnum<file>, error out=w121:errorcluster)  [unwired: 4 in, 1 out]
              n115 = Close File(refnum=w122, error in=w121) -> (error out=w117:errorcluster)  [unwired: 1 out]
              n116 = call <vilib>:"Check if File or Folder Exists.vi"("error in (no error)"=w117, "path"=path "C:/Users/Admin/Documents/Automation_Tests/communication.txt" ("file (use dialog)")) -> ("file or folder exists?"=w118:bool)  [unwired: 7 in, 2 out]
            }
          }
          frame #2 {
            n117 = Wait (ms)(milliseconds to wait=u32 500) -> ()  [unwired: 1 out]
          }
          frame #3 {
            n118 = global write "DAQGlobal.vi" "Saving?"(TRUE ("Saving?")) -> ()
          }
          frame #4 {
            n119 = local read "Exposure Time:"() -> (w128:dbl)
            n120 = Multiply(x=w128, y=1000.0) -> (x*y=w126:dbl)
            n121 = Wait (ms)(milliseconds to wait=w126) -> ()  [unwired: 1 out]
          }
          frame #5 {
            n122 = global write "DAQGlobal.vi" "Saving?"(FALSE ("Saving?")) -> ()
          }
          frame #6 {
            n123 = while {
              stop <- w131 continue-if-true
              n124 = call <vilib>:"Check if File or Folder Exists.vi"("path"=path "C:/Users/Admin/Documents/Automation_Tests/communication.txt" ("file (use dialog)")) -> ("file or folder exists?"=w131:bool)  [unwired: 8 in, 2 out]
              n125 = Wait (ms)(milliseconds to wait=u32 100) -> ()  [unwired: 1 out]
            }
          }
          frame #7 {
          }
        }
        n126 = disable-structure shown="Enabled" {
          disable-tunnel: [w114 TRUE] -> w111
          frame #0 {
            w114 = TRUE
            n127 = global write "DAQGlobal.vi" "Saving?"(w114) -> ()
          }
          frame #1 {
          }
        }
      }
      frame #4 {
        # "Probably Not"
        # "This may \nbe broken?"
        n128 = flat-sequence {
          tunnel: [autostatus."Next Wavelength" ("Auto Status")] -> w134
          frame #0 {
            n129 = Wait (ms)(milliseconds to wait=u32 1000) -> ()  [unwired: 1 out]
          }
          frame #1 {
            n130 = while {
              stop <- w142 stop-if-true
              n131 = Open/Create/Replace File(file path (use dialog)=path "C:/Users/Admin/Documents/Automation_Tests/communication.txt" ("file (use dialog)"), operation (0:open)=T1."replace or create") -> (refnum out=w146:refnum<file>, error out=w145:errorcluster)  [unwired: 4 in, 1 out]
              n132 = Close File(refnum=w146, error in=w145) -> (error out=w141:errorcluster)  [unwired: 1 out]
              n133 = call <vilib>:"Check if File or Folder Exists.vi"("error in (no error)"=w141, "path"=path "C:/Users/Admin/Documents/Automation_Tests/communication.txt" ("file (use dialog)")) -> ("file or folder exists?"=w142:bool)  [unwired: 7 in, 2 out]
            }
          }
          frame #2 {
            n134 = Wait (ms)(milliseconds to wait=u32 500) -> ()  [unwired: 1 out]
          }
          frame #3 {
            n135 = global write "DAQGlobal.vi" "Saving?"(TRUE ("Saving?")) -> ()
          }
          frame #4 {
            n136 = local read "Exposure Time:"() -> (w152:dbl)
            n137 = Multiply(x=w152, y=1000.0) -> (x*y=w150:dbl)
            n138 = Wait (ms)(milliseconds to wait=w150) -> ()  [unwired: 1 out]
          }
          frame #5 {
            n139 = global write "DAQGlobal.vi" "Saving?"(FALSE ("Saving?")) -> ()
          }
          frame #6 {
            n140 = while {
              stop <- w155 continue-if-true
              n141 = call <vilib>:"Check if File or Folder Exists.vi"("path"=path "C:/Users/Admin/Documents/Automation_Tests/communication.txt" ("file (use dialog)")) -> ("file or folder exists?"=w155:bool)  [unwired: 8 in, 2 out]
              n142 = Wait (ms)(milliseconds to wait=u32 100) -> ()  [unwired: 1 out]
            }
          }
          frame #7 {
          }
        }
        n143 = disable-structure shown="Enabled" {
          disable-tunnel: [w138 TRUE] -> w135
          frame #0 {
            w138 = TRUE
            n144 = global write "DAQGlobal.vi" "Saving?"(w138) -> ()
          }
          frame #1 {
          }
        }
      }
      frame #5 {
        # "Used to be Next WL"
      }
      frame #6 {
        n145 = local read "Present Wavelength"() -> (w167:dbl)
        n146 = local read "Max nm"() -> (w170:dbl)
        n147 = Greater Or Equal?(x=w167, y=w170) -> (x >= y?=w169:bool)
        n148 = case shown="False" w169 {
          tunnel: [w181 w184] -> w168
          tunnel: w167 -> [w178 _]
          tunnel: [TRUE ("Waiting on Move") FALSE ("Waiting on Move")] -> w166
          tunnel: w165 -> [_ w184]
          tunnel: [autostatus."Default" ("Auto Status") autostatus."Default" ("Auto Status")] -> w164
          tunnel: w163 -> [w172 w182]
          tunnel: [w171 w182] -> w162
          frame #0 {
            n149 = local read "Calibration, nm"() -> (w177:dbl)
            n150 = local read "Grating, gr/mm"() -> (w176:u16)
            n151 = local write "Waiting on Move"(TRUE ("Waiting on Move")) -> ()
            n152 = local read "Step Size:"() -> (w180:dbl)
            n153 = Add(x=w178, y=w180) -> (x+y=w179:dbl)
            "GoTo Wavelength" <- w179
            n154 = call "wavelength_string.vi"("error in (no error)"=w172, "Grating, gr/mm"=w176, "Destination Wavelength"=w179, "Calibration, nm"=w177) -> ("error out"=w171:errorcluster, "Wavelength_String"=w181:string)
          }
          frame #1 {
          }
        }
      }
    }
    "command sent" <- w42
    "writing" <- w33
    n155 = case shown="True" w33 {
      tunnel: "Delay Before\nread (ms)" -> [w203 w209]
      tunnel: [w193 w214] -> w36
      tunnel: [w204 w213] -> w37
      tunnel: w42 -> [_ w208]
      tunnel: w44 -> [w197 w207]
      tunnel: w29 -> [w196 w206]
      tunnel: [w195 w205] -> w34
      tunnel: w32 -> [_ w205]
      frame #0 {
        w201 = TRUE ("write")
        n156 = local read "Calibration, nm"() -> (w198:dbl)
        n157 = local read "Grating, gr/mm"() -> (w199:u16)
        n158 = call "RS232.vi"("read"=w201, "delay before read (ms)"=w203, "error in"=w196, "write"=w201, "string to write"="X-1?", "VISA  name in"=w197) -> ("error out"=w194:errorcluster, "read string"=w200:string, "VISA out"=w204:refnum<visa-resource-name>)  [unwired: 1 out]
        "string 2" <- w200
        n159 = call "string_wavelength.vi"("error in (no error)"=w194, "Grating, gr/mm"=w199, "Position String"=w200, "Calibration, nm"=w198) -> ("error out"=w193:errorcluster, "Present Wavelength"=w195:dbl)
        "Present Wavelength" <- w195
      }
      frame #1 {
        w215 = TRUE ("write")
        n160 = call "RS232.vi"("read"=w215, "delay before read (ms)"=w209, "error in"=w206, "write"=w215, "string to write"=w208, "VISA  name in"=w207) -> ("error out"=w214:errorcluster, "read string"=w212:string, "VISA out"=w213:refnum<visa-resource-name>)  [unwired: 1 out]
        "read string" <- w212
        n161 = call "string_winding_state_probe_ON.vi"("read string"=w212) -> ("ON"=→"Shutter ON":bool)
        n162 = call "string_winding_state_probe_OFF.vi"("read string"=w212) -> ("OFF"=→"Shutter OFF":bool)
      }
    }
    n163 = Unbundle By Name(w36) -> ("status"=w63:bool)
    n164 = Select(t=w32, s=w33, f=w34) -> (s? t:f=w35:dbl)
    n165 = Or(x=w63, y="stop") -> (x .or. y?=w61:bool)
    "Loop" <- w68
  }
  n166 = VISA Close(VISA resource name=w6, error in (no error)=w7) -> (error out=w10:errorcluster)
  n167 = call <vilib>:"Simple Error Handler.vi"("error in (no error)"=w10) -> ("error out"=w5:errorcluster)  [unwired: 4 in, 4 out]
  n168 = Open/Create/Replace File(file path (use dialog)=path "C:/Users/Admin/Documents/Automation_Tests/shutdown.txt", error in=w5, operation (0:open)=T1."replace or create") -> (refnum out=w1:refnum<file>, error out=w2:errorcluster)  [unwired: 3 in, 1 out]
  n169 = Close File(refnum=w1, error in=w2) -> ()  [unwired: 2 out]
